vi "Pairwise_kernels.vi"(8 "error in":errorcluster caption="entrée d'erreur", 9 "Y":string[][](array[string]), 10 "X":string[][](array[string]), 11 "pairwise_kernels":T2={"metric "="linear", "filter_params"=FALSE, "n_jobs"="None"}) -> (0 "error out":errorcluster caption="sortie d'erreur", 3 "Data":T1)   [LabVIEW 2020]
doc: "Compute the kernel between arrays X and optional array Y.\n\nThis method takes either a vector array or a kernel matrix, and returns a kernel matrix. If the input is a vector array, the kernels are computed. If the input is a kernel matrix, it is returned instead.\n\nThis method provides a safe way to take a kernel matrix as input, while preserving compatibility with many other algorithms that take a vector array.\n\nIf Y is given (default is None), then the returned matrix is the pairwise kernel between the arrays from both X and Y.\n\nValid values for metric are :\n\n [‘additive_chi2’, ‘chi2’, ‘linear’, ‘poly’, ‘polynomial’, ‘rbf’, ‘laplacian’, ‘sigmoid’, ‘cosine’]\n\n\nParameters :\n\n- X : array [n_samples_a, n_samples_a] if metric == “precomputed”, or, [n_samples_a, n_features] otherwise\nArray of pairwise kernels between samples, or a feature array.\n\n- Y : array [n_samples_b, n_features]\nA second feature array only if X has shape [n_samples_a, n_features].\n\n- metric : string, or callable\nThe metric to use when calculating kernel between instances in a feature array. If metric is a string, it must be one of the metrics in pairwise.PAIRWISE_KERNEL_FUNCTIONS. If metric is “precomputed”, X is assumed to be a kernel matrix. Alternatively, if metric is a callable function, it is called on each pair of instances (rows) and the resulting value recorded. The callable should take two rows from X as input and return the corresponding kernel value as a single number. This means that callables from sklearn.metrics.pairwise are not allowed, as they operate on matrices, not single samples. Use the string identifying the kernel instead.\n\n- filter_params : boolean\nWhether to filter invalid parameters or not.\n\n- n_jobs : int or None, optional (default=None)\nThe number of jobs to use for the computation. This works by breaking down the pairwise matrix into n_jobs even slices and computing them in parallel.\n\nNone means 1 unless in a joblib.parallel_backend context. -1 means using all processors. See Glossary for more details.\n\n\nReturns : \n\n- K : array [n_samples_a, n_samples_a] or [n_samples_a, n_samples_b]\nA kernel matrix K such that K_{i, j} is the kernel between the ith and jth vectors of the given matrix X, if Y is None. If Y is not None, then K_{i, j} is the kernel between the ith array from X and the jth array from Y."
uses:
  Pairwise_kernels.lvclass
panel:
  out "Pairwise_kernels.lvclass":refnum<class "Pairwise_kernels.lvclass">
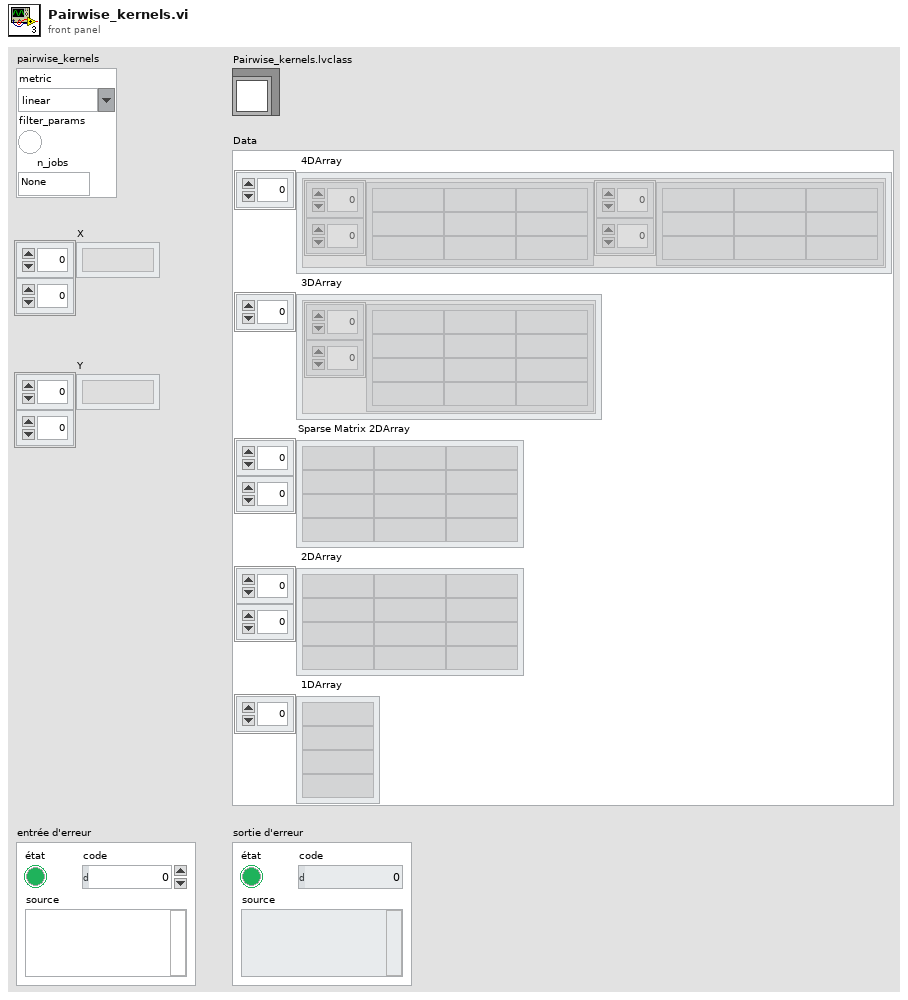
[diagram p1: front panel]
types:
  T1 = cluster{" 4DArray":cluster{"1":string[][], "2":string[][]}[], " 3DArray":cluster{"Tableau":string[][]}[], "Sparse Matrix 2DArray":string[][], " 2DArray":string[][], " 1DArray":string[]}
  T2 = cluster{"metric ":string, "filter_params":bool, "n_jobs":string}
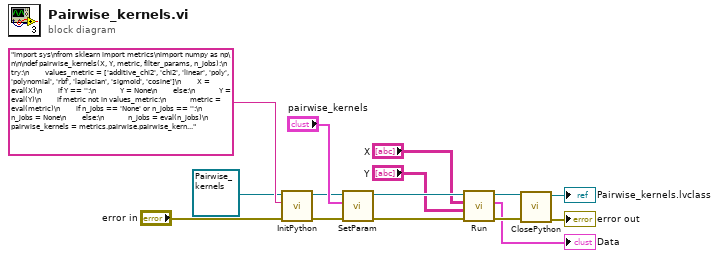
[diagram p0: block diagram]
diagram:
  n1 = call-dynamic "InitPython.vi"("error in (no error)"="error in", "Python Instruction"="import sys\nfrom sklearn import metrics\nimport numpy as np\n\n\ndef pairwise_kernels(X, Y, metric, filter_params, n_jobs):\n    try:\n        values_metric = ['additive_chi2', 'chi2', 'linear', 'poly', 'polynomial', 'rbf', 'laplacian', 'sigmoid', 'cosine']\n        X = eval(X)\n        if Y == '':\n            Y = None\n        else:\n            Y = eval(Y)\n        if metric not in values_metric:\n            metric = eval(metric)\n        if n_jobs == 'None' or n_jobs == '':\n            n_jobs = None\n        else:\n            n_jobs = eval(n_jobs)\n        pairwise_kernels = metrics.pairwise.pairwise_kernels(X, Y, metric, filter_params, n_jobs)\n        pairwise_kernels = pairwise_kernels.tolist()\n        return str(pairwise_kernels)\n    except:\n        erreur = sys.exc_info()\n        typerr = u\"%s\" % (erreur[0])\n        typerr = typerr[typerr.find(\"'\")+1:typerr.rfind(\"'\")]\n        msgerr = u\"%s\" % (erreur[1])\n        message = str('/!\\\\ {0} : {1}'. format(typerr,msgerr))\n        return message", "Scikit-learn en entrée"=refnum<class "Pairwise_kernels.lvclass"> refnum ("Pairwise_kernels.lvclass")) -> ("error out"=w13:errorcluster, "Scikit-learn en sortie"=w11:refnum<class "Pairwise_kernels.lvclass">)  [unwired: 7 in]
  n2 = call-dynamic "SetParam.vi"("error in (no error)"=w13, "pairwise_kernels"="pairwise_kernels", "Pairwise_kernels.lvclass"=w11) -> ("error out"=w9:errorcluster, "Pairwise_kernels.lvclass"=w10:refnum<class "Pairwise_kernels.lvclass">)  [unwired: 7 in]
  n3 = call-dynamic "Run.vi"("error in (no error)"=w9, "Y"="Y", "X"="X", "Pairwise_kernels.lvclass"=w10) -> ("error out"=w7:errorcluster, "Data"=→"Data":T1, "Pairwise_kernels.lvclass"=w8:refnum<class "Pairwise_kernels.lvclass">)  [unwired: 5 in]
  n4 = call-dynamic "ClosePython.vi"("error in (no error)"=w7, "Scikit-learn en entrée"=w8) -> ("error out"=→"error out":errorcluster, "Scikit-learn en sortie"=→"Pairwise_kernels.lvclass":refnum<class "Pairwise_kernels.lvclass">)  [unwired: 8 in]
